vi "AudioTest.Read Single Plot Definition File.vi"(8 "error in (no error)":errorcluster, 11 "CSV File":path) -> (0 "error out":errorcluster, 3 "Plot":T1)   [LabVIEW 2018]
uses:
  TypeDefs/AudioTest.Result Plot Data.ctl
  <vilib>/KATE/Files/File Utils.lvlib
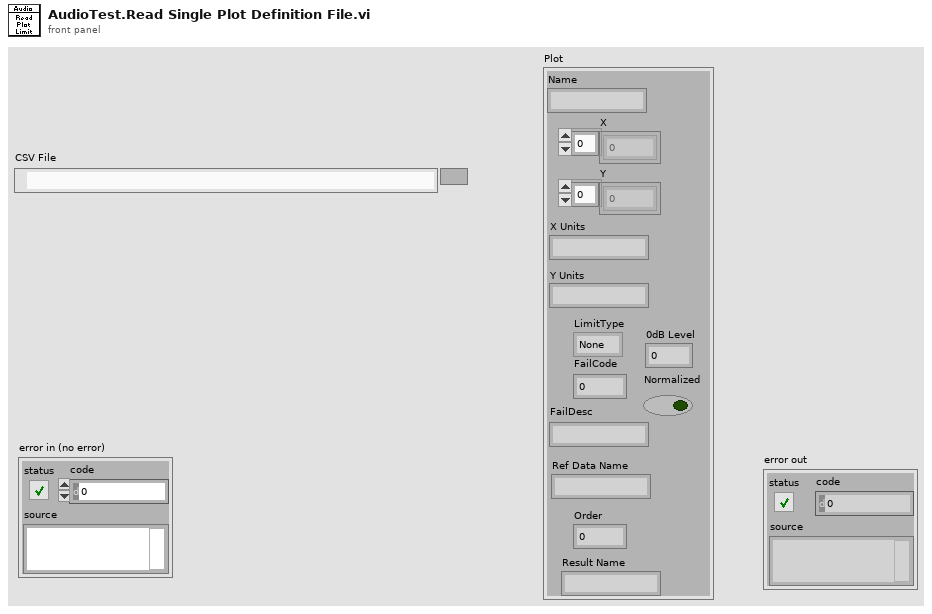
[diagram p1: front panel]
types:
  T1 = typedef "AudioTest.Result Plot Data.ctl" = cluster{"Order":i32, "Name":string, "X":dbl[], "Y":dbl[], "X Units":string, "Y Units":string, "LimitType":enum16{"None", "LL", "UL"}, "FailCode":i32, "FailDesc":string, "Ref Data Name":string, "Result Name":string, "0dB Level":dbl, "Normalized":bool}
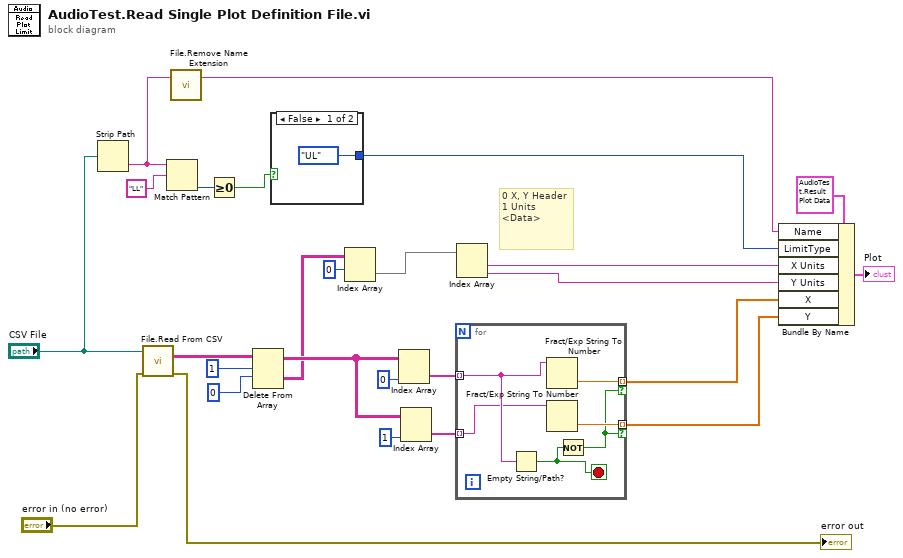
[diagram p0: block diagram]
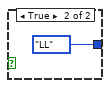
[diagram p2: hidden frame]
diagram:
  # "0 X, Y Header\n1 Units\n<Data>"
  n1 = Strip Path(path="CSV File") -> (name=w6:string)  [unwired: 1 out]
  n2 = call <vilib>:"File.Read From CSV.vi"("error in"="error in (no error)", "File"="CSV File") -> ("error out"=→"error out":errorcluster, "Data"=w26:string[][])  [unwired: 7 in, 1 out]
  n3 = Match Pattern(string=w6, regular expression="LL") -> (offset past match=w9:i32)  [unwired: 1 in, 3 out]
  n4 = call <vilib>:"File.Remove Name Extension.vi"("File Name"=w6) -> ("Name Less Ext"=w5:string)  [unwired: 1 in, 1 out]
  n5 = Greater Or Equal To 0?(x=w9) -> (x >= 0?=w8:bool)
  n6 = Delete From Array(array=w26, length=1, index (row)=0) -> (deleted portion=w15:string[][], array with subset deleted=w20:string[][])  [unwired: 1 in]
  n7 = case shown="False" w8 {
    tunnel: [enum16{"None", "LL", "UL"}."UL" ("LimitType") enum16{"None", "LL", "UL"}."LL" ("LimitType")] -> w4
    frame False {
    }
    frame True {
    }
  }
  n8 = Index Array(array=w15, index (row)=0) -> (element=w13:string[])  [unwired: 1 in]
  n9 = Index Array(array=w20, index (col)=0 ("disabled index (col)")) -> (element=w19:string[])  [unwired: 1 in]
  n10 = Index Array(array=w20, index (col)=1 ("disabled index (col)")) -> (element=w18:string[])  [unwired: 1 in]
  n11 = for {
    tunnel: w19 -> [w34] mode=indexing
    tunnel: w18 -> [w33] mode=indexing
    tunnel: [w32] -> w7 mode=indexing if=w29
    tunnel: [w31] -> w3 mode=indexing if=w29
    stop <- w30 stop-if-true
    n12 = Empty String/Path?(string/path=w34) -> (empty?=w30:bool)
    n13 = Fract/Exp String To Number(string=w34) -> (number=w31:dbl)  [unwired: 3 in, 1 out]
    n14 = Fract/Exp String To Number(string=w33) -> (number=w32:dbl)  [unwired: 3 in, 1 out]
    n15 = Not(x=w30) -> (.not. x?=w29:bool)
  }
  n16 = Index Array(array=w13) -> (element #1=w16:string, element #2=w17:string)  [unwired: 2 in]
  n17 = Bundle By Name(cluster=T1 {"Order"=0, "Name"="", "X"=[], "Y"=[], "X Units"="", "Y Units"="", "LimitType"=enum."None", "FailCode"=0, "FailDesc"="", "Ref Data Name"="", "Result Name"="", "0dB Level"=0.0, "Normalized"=FALSE}, "Name"=w5, "LimitType"=w4, "X Units"=w16, "Y Units"=w17, "X"=w3, "Y"=w7) -> (→"Plot":T1)
